vi "Scilab+Labview.vi"() -> ()   [LabVIEW 2015]
panel:
  in  "stop":bool
  out "Real 2":dbl
  out "error out":errorcluster
  in  "Real":dbl
  in  "error in":errorcluster
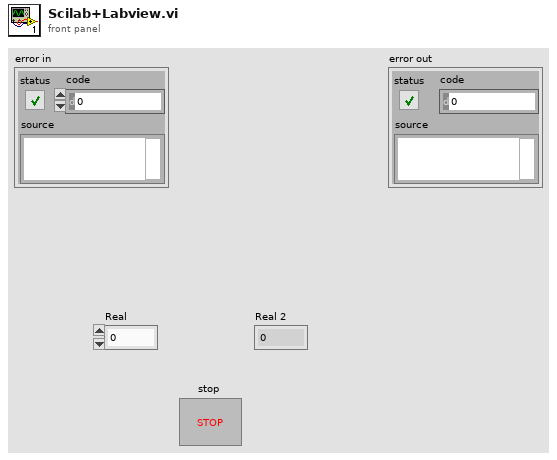
[diagram p1: front panel]
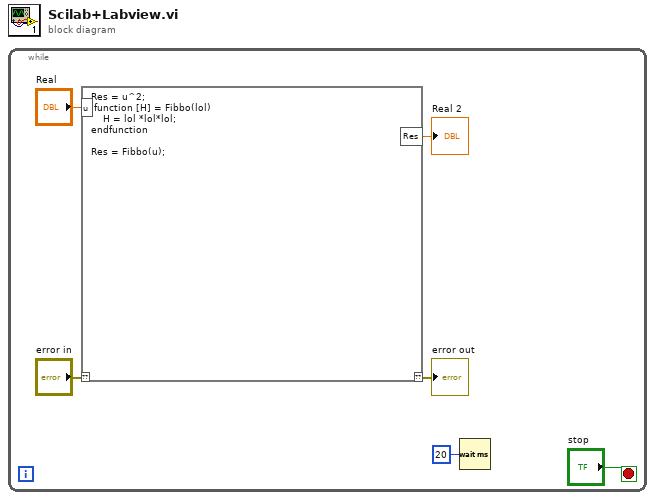
[diagram p0: block diagram]
diagram:
  n1 = while {
    stop <- "stop" stop-if-true
    n2 = script code="Res = u^2;\n function [H] = Fibbo(lol)\n    H = lol *lol*lol;\nendfunction\n\nRes = Fibbo(u);"("??"="error in", "u"="Real") -> ("??"=→"error out":errorcluster, "Res"=→"Real 2":dbl)
    n3 = Wait (ms)(milliseconds to wait=u32 20) -> ()  [unwired: 1 out]
  }
